vi "LED State.vi"() -> ()   [LabVIEW 2015]
panel:
  in  "LED State":bool
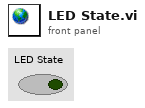
[diagram p1: front panel]
diagram:
